vi "zmq REQ.vi"() -> ()   [LabVIEW 2018]
uses:
  <vilib>/addons/zeromq/poll_type.ctl
  <vilib>/addons/zeromq/socket_type.ctl
  <vilib>/addons/zeromq/zmq_context.lvclass
  <vilib>/addons/zeromq/zeromq.lvlib
  <vilib>/addons/zeromq/zmq_socket.lvclass
panel:
  in  "Connection Type":enum16{"connect", "bind"}(ring)
  in  "Poll":bool
  out "timed out?":bool
  out "nevents":i32
  out "polled events":T1[](array[typedef])
  in  "poll type":T1=enum."In/Out"
  in  "receive":bool
  in  "Message":string="{\"msg_id\":\"555\",\"msg_type\":\"read\",\"msg_property\":\"vmon\",\"8-04\":\"XXX\"}"
  in  "SEND":bool
  out "HB":bool
  out "error out":errorcluster
  in  "stop":bool
  in  "ZMQ endpoint":string="tcp://127.0.0.1:5555"
  out "REPLY":string
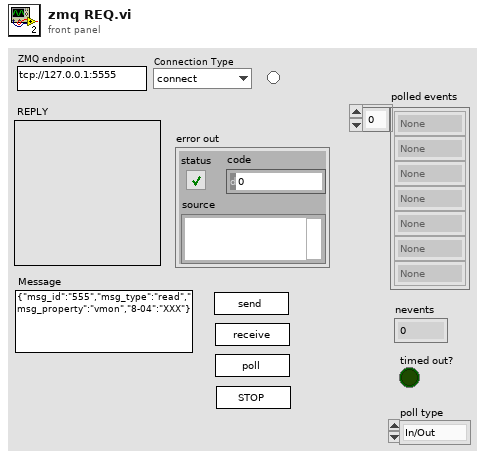
[diagram p1: front panel]
types:
  T1 = typedef "zeromq.lvlib/poll_type.ctl" = enum16{"None", "In", "Out", "In/Out"}
  T2 = typedef "zeromq.lvlib/socket_type.ctl" = enum8{"ZMQ_PAIR", "ZMQ_PUB", "ZMQ_SUB", "ZMQ_REQ", "ZMQ_REP", "ZMQ_DEALER", "ZMQ_ROUTER", "ZMQ_PULL", "ZMQ_PUSH", "ZMQ_XPUB", "ZMQ_XSUB"}
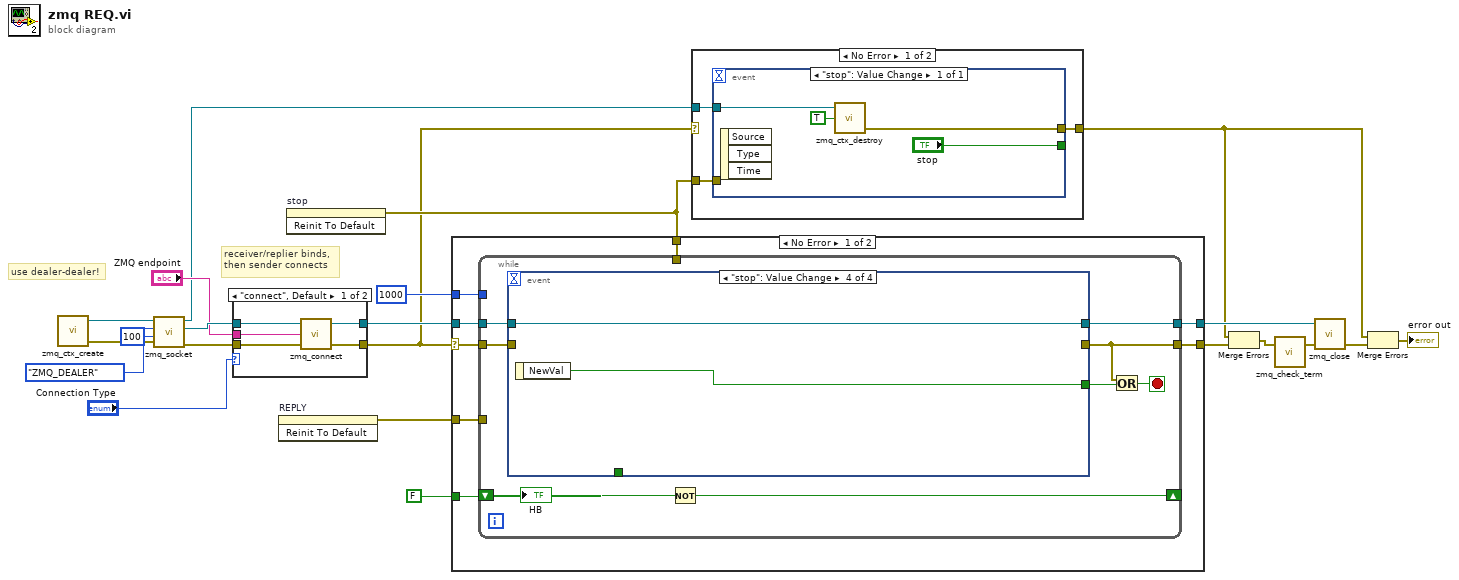
[diagram p0: block diagram]
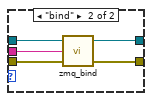
[diagram p2: hidden frame]
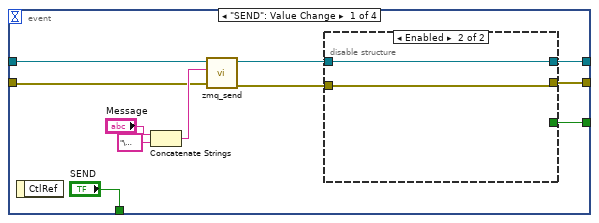
[diagram p3: hidden frame]
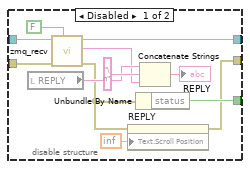
[diagram p4: hidden frame]
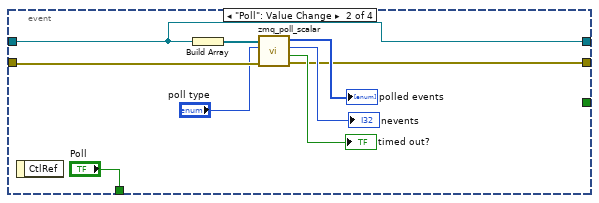
[diagram p5: hidden frame]
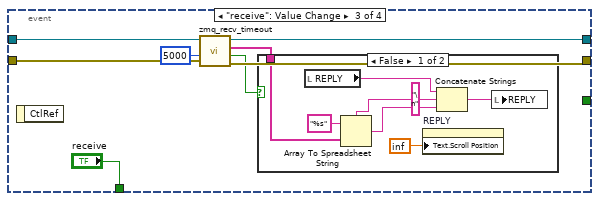
[diagram p6: hidden frame]
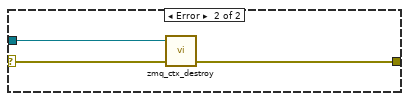
[diagram p9: hidden frame]
diagram:
  # "receiver/replier binds,\nthen sender connects"
  # "use dealer-dealer!"
  n1 = call <vilib>:"zmq_ctx_create.vi"() -> ("error out"=w15:errorcluster, "context out"=w13:refnum<class "zmq_context.lvclass">)  [unwired: 4 in]
  n2 = call <vilib>:"zmq_socket.vi"("error in"=w15, "linger (ms)"=100, "socket type"=socket_type."ZMQ_DEALER", "context in"=w13) -> ("error out"=w20:errorcluster, "socket out"=w21:refnum<class "zmq_socket.lvclass">, "context out"=w4:refnum<class "zmq_context.lvclass">)  [unwired: 1 in]
  n3 = case shown="\"connect\", Default" "Connection Type" {
    tunnel: w21 -> [w27 w32]
    tunnel: w20 -> [w26 w29]
    tunnel: [w25 w31] -> w19
    tunnel: "ZMQ endpoint" -> [w24 w28]
    tunnel: [w23 w30] -> w6
    frame "connect", Default {
      n4 = call <vilib>:"zmq_connect.vi"("error in"=w26, "endpoint"=w24, "socket in"=w27) -> ("error out"=w23:errorcluster, "socket out"=w25:refnum<class "zmq_socket.lvclass">)  [unwired: 1 in]
    }
    frame "bind" {
      n5 = call <vilib>:"zmq_bind.vi"("error in"=w29, "endpoint"=w28, "socket in"=w32) -> ("error out"=w30:errorcluster, "socket out"=w31:refnum<class "zmq_socket.lvclass">)  [unwired: 1 in]
    }
  }
  n6 = invoke on="REPLY" class="Str" method="Reinit To Default"() -> (error out=w14:errorcluster)  [unwired: 3 in, 2 out]
  n7 = invoke on="stop" class="Bool" method="Reinit To Default"() -> (error out=w8:errorcluster)  [unwired: 3 in, 2 out]
  n8 = case shown="No Error" w6 {
    selector: w6 -> [w33 w101]
    tunnel: w19 -> [w40 w100]
    tunnel: 1000 -> [w39 _]
    tunnel: [w38 w100] -> w17
    tunnel: w14 -> [w37 _]
    tunnel: [w36 w101] -> w3
    tunnel: FALSE ("stop") -> [w35 _]
    tunnel: w8 -> [w34 _]
    frame No Error {
      n9 = while {
        tunnel: w40 -> [w48]
        tunnel: w33 -> [w47]
        tunnel: w39 -> [_]
        tunnel: [w46] -> w38
        tunnel: [w41] -> w36
        tunnel: w37 -> [_]
        shift-right: [w44] -> _
        shift-left: w35 -> [w45]
        tunnel: w34 -> [_]
        stop <- w43 stop-if-true
        n10 = event shown="[3] \"stop\": Value Change" {
          selector: _ -> [_ _ _ _]
          dyn-events: _ -> [_ _ _ _]
          timeout: _ -> [_ _ _ _]
          tunnel: [w58 _ _ w98] -> w42
          tunnel: w48 -> [w49 w76 w90 w99]
          tunnel: w47 -> [w50 w77 w89 _]
          tunnel: [w57 w76 w86 w99] -> w46
          tunnel: [w51 w75 w87 _] -> w41
          tunnel: ["SEND" "Poll" "receive" _] -> _
          event "SEND": Value Change {
            n11 = event-data() -> ()  [unwired: 1 in, 1 out]
            n12 = Concatenate Strings("Message", "\u0000" ("string")) -> (w52:string)
            n13 = call <vilib>:"zmq_send.vi"("error in"=w50, "data"=w52, "socket in"=w49) -> ("error out"=w56:errorcluster, "socket out"=w59:refnum<class "zmq_socket.lvclass">)  [unwired: 4 in]
            n14 = disable-structure shown="Enabled" {
              disable-tunnel: w59 -> [w71 w73]
              disable-tunnel: [w70 _] -> w58
              disable-tunnel: [w69 w73] -> w57
              disable-tunnel: w56 -> [w67 w72]
              disable-tunnel: [w60 w72] -> w51
              frame Disabled {
                n15 = local read "REPLY"() -> (w63:string)
                n16 = call <vilib>:"zmq_recv.vi"("no block? (F)"=FALSE, "error in"=w67, "socket in"=w71) -> ("error out"=w61:errorcluster, "data"=w62:string, "socket out"=w69:refnum<class "zmq_socket.lvclass">)  [unwired: 2 in, 2 out]
                n17 = property on="REPLY" class="Str"(error in=w61, "Text.Scroll Position"=inf) -> (error out=w60:errorcluster)  [unwired: 1 in, 1 out]
                n18 = Unbundle By Name(w61) -> ("status"=w70:bool)
                n19 = Concatenate Strings(w63, "\n" ("string"), w62) -> (→"REPLY":string)
              }
              frame Enabled {
              }
            }
          }
          event "Poll": Value Change {
            n20 = event-data() -> ()  [unwired: 1 in, 1 out]
            n21 = Build Array(w76) -> (w81:refnum<class "zmq_socket.lvclass">[])
            n22 = call <vilib>:"zmq_poll_scalar.vi"("error in"=w77, "poll type"="poll type", "sockets"=w81) -> ("error out"=w75:errorcluster, "timed out?"=→"timed out?":bool, "nevents"=→"nevents":i32, "polled events"=→"polled events":T1[])  [unwired: 1 in]
          }
          event "receive": Value Change {
            n23 = event-data() -> ()  [unwired: 1 in, 1 out]
            n24 = call <vilib>:"zmq_recv_timeout.vi"("error in"=w89, "timeout (ms)"=u32 5000, "socket in"=w90) -> ("error out"=w87:errorcluster, "timeout?"=w84:bool, "parts"=w85:string[], "socket out"=w86:refnum<class "zmq_socket.lvclass">)  [unwired: 1 in]
            n25 = case shown="False" w84 {
              tunnel: w85 -> [w93 _]
              frame False {
                w94 = "\n" ("string")
                n26 = local read "REPLY"() -> (w96:string)
                n27 = Array To Spreadsheet String(delimiter (Tab)=w94, array=w93, 3:"%s" ("format string")) -> (spreadsheet string=w92:string)
                n28 = property on="REPLY" class="Str"("Text.Scroll Position"=inf) -> ()  [unwired: 2 in, 2 out]
                n29 = Concatenate Strings(w96, w94, w92) -> (w97:string)
                n30 = local write "REPLY"(w97) -> ()
              }
              frame True {
              }
            }
          }
          event "stop": Value Change {
            n31 = event-data() -> ("NewVal"=w98:bool)  [unwired: 1 in]
          }
        }
        n32 = Not(x=w45) -> (.not. x?=w44:bool)
        n33 = Or(x=w41, y=w42) -> (x .or. y?=w43:bool)
        "HB" <- w45
      }
    }
    frame Error {
    }
  }
  n34 = case shown="No Error" w6 {
    selector: w6 -> [_ w110]
    tunnel: w4 -> [w104 w111]
    tunnel: [w103 w109] -> w1
    tunnel: w8 -> [w102 _]
    frame No Error {
      n35 = event shown="[0] \"stop\": Value Change" {
        selector: _ -> [_]
        dyn-events: _ -> [_]
        timeout: _ -> [_]
        tunnel: w104 -> [w108]
        tunnel: ["stop"] -> _
        tunnel: [w106] -> w103
        tunnel: w102 -> [_]
        event "stop": Value Change {
          n36 = event-data() -> ()  [unwired: 1 in, 3 out]
          n37 = call <vilib>:"zmq_ctx_destroy.vi"("reap? (F)"=TRUE, "context in"=w108) -> ("error out"=w106:errorcluster)  [unwired: 3 in]
        }
      }
    }
    frame Error {
      n38 = call <vilib>:"zmq_ctx_destroy.vi"("error in"=w110, "context in"=w111) -> ("error out"=w109:errorcluster)  [unwired: 3 in]
    }
  }
  n39 = Merge Errors(w1, w3) -> (w2:errorcluster)
  n40 = call <vilib>:"zmq_check_term.vi"("error in"=w2) -> ("error out"=w12:errorcluster)  [unwired: 1 in, 1 out]
  n41 = call <vilib>:"zmq_close.vi"("error in"=w12, "socket"=w17) -> ("error out"=w11:errorcluster)  [unwired: 3 in]
  n42 = Merge Errors(w1, w11) -> (→"error out":errorcluster)
